vi "ShooterSpeedRegulateV1.vi"(0 "Shooter Speed":T1(ring)) -> (4 "ALL GOOD":bool, 10 "Motor 1 Output":dbl)   [LabVIEW 2012]
uses:
  Robot Global Data.vi
  Max'sToolKit/ConvertVoltageToPercentVbs.vi
  <vilib>/addons/control/pid/pid.llb/PID (DBL).vi
  <vilib>/addons/control/pid/NI_PID_pid.lvlib
panel:
  in  "Reset Shooter PID":bool
  out "Loop Rate (Hz)":dbl
  out "Array Index":dbl
  out "Wheel 1 RPS":dbl
  out "W1 Target RPS":dbl
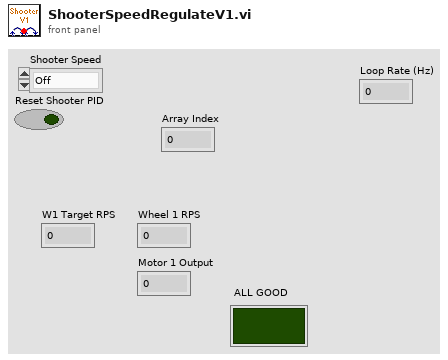
[diagram p1: front panel]
types:
  T1 = enum16{"Off", "2pt Key Shot", "3pt Key Shot", "Back Shot", "Fender Shot", "Key Close", "Key Far"}
  T2 = typedef "WPI_EncoderDevRef.ctl" = cluster{"DevStatus":errorcluster, "EncoderIndex":T3, "CounterIndex":T4, "DistancePerCount":dbl, "Decoding Type":T5}
  T3 = typedef "FPGA_EncoderIdx.ctl" = enum8{"Enc 0", "Enc 1", "Enc 2", "Enc 3", "Invalid"}
  T4 = typedef "FPGA_CounterCtrSystemIndex.ctl" = enum8{"Ctr 0", "Ctr 1", "Ctr 2", "Ctr 3", "Ctr 4", "Ctr 5", "Ctr 6", "Ctr 7", "Invalid"}
  T5 = typedef "WPI_EncoderType.ctl" = enum16{"1x", "2x", "4x"}
  T6 = cluster{"proportional gain (Kc)":dbl, "integral time (Ti, min)":dbl, "derivative time (Td, min)":dbl}
  T7 = typedef "WPI_MotorControlDeviceRef.ctl" = cluster{"DeviceStatus":errorcluster, "Type":enum16{"PWM", "CAN"}, "PWM":cluster{"Digital Module":T8, "PWM Channel":T9, "DeadBand":T10}, "CAN":cluster{"Device Number":u8, "Control Mode":T11, "Semaphore":T12, "Max Vout":dbl}, "Invert":bool, "TransformRef":T13, "InvTransformRef":T13}
  T8 = typedef "FPGA_TypedefDigitalModule.ctl" = enum16{"Digital Module 1", "Digital Module 2"}
  T9 = typedef "FPGA_DIOPWMChannel.ctl" = enum8{"PWM 1", "PWM 2", "PWM 3", "PWM 4", "PWM 5", "PWM 6", "PWM 7", "PWM 8", "PWM 9", "PWM 10", "Invalid"}
  T10 = typedef "WPI_PWMDeadband.ctl" = cluster{"Name":string, "maxPositivePwm":i32, "minPositivePwm":i32, "centerPwm":i32, "maxNegativePwm":i32, "minNegativePwm":i32, "angularRange":u16}
  T11 = typedef "WPI_CANJaguar_ControlMode.ctl" = enum8{"Percent VBus", "Current", "Speed", "Position", "Voltage"}
  T12 = typedef "Semaphore RefNum" = refnum<k1>
  T13 = typedef "WPI_PWMTransform_ConPane.ctl" = refnum<vi>
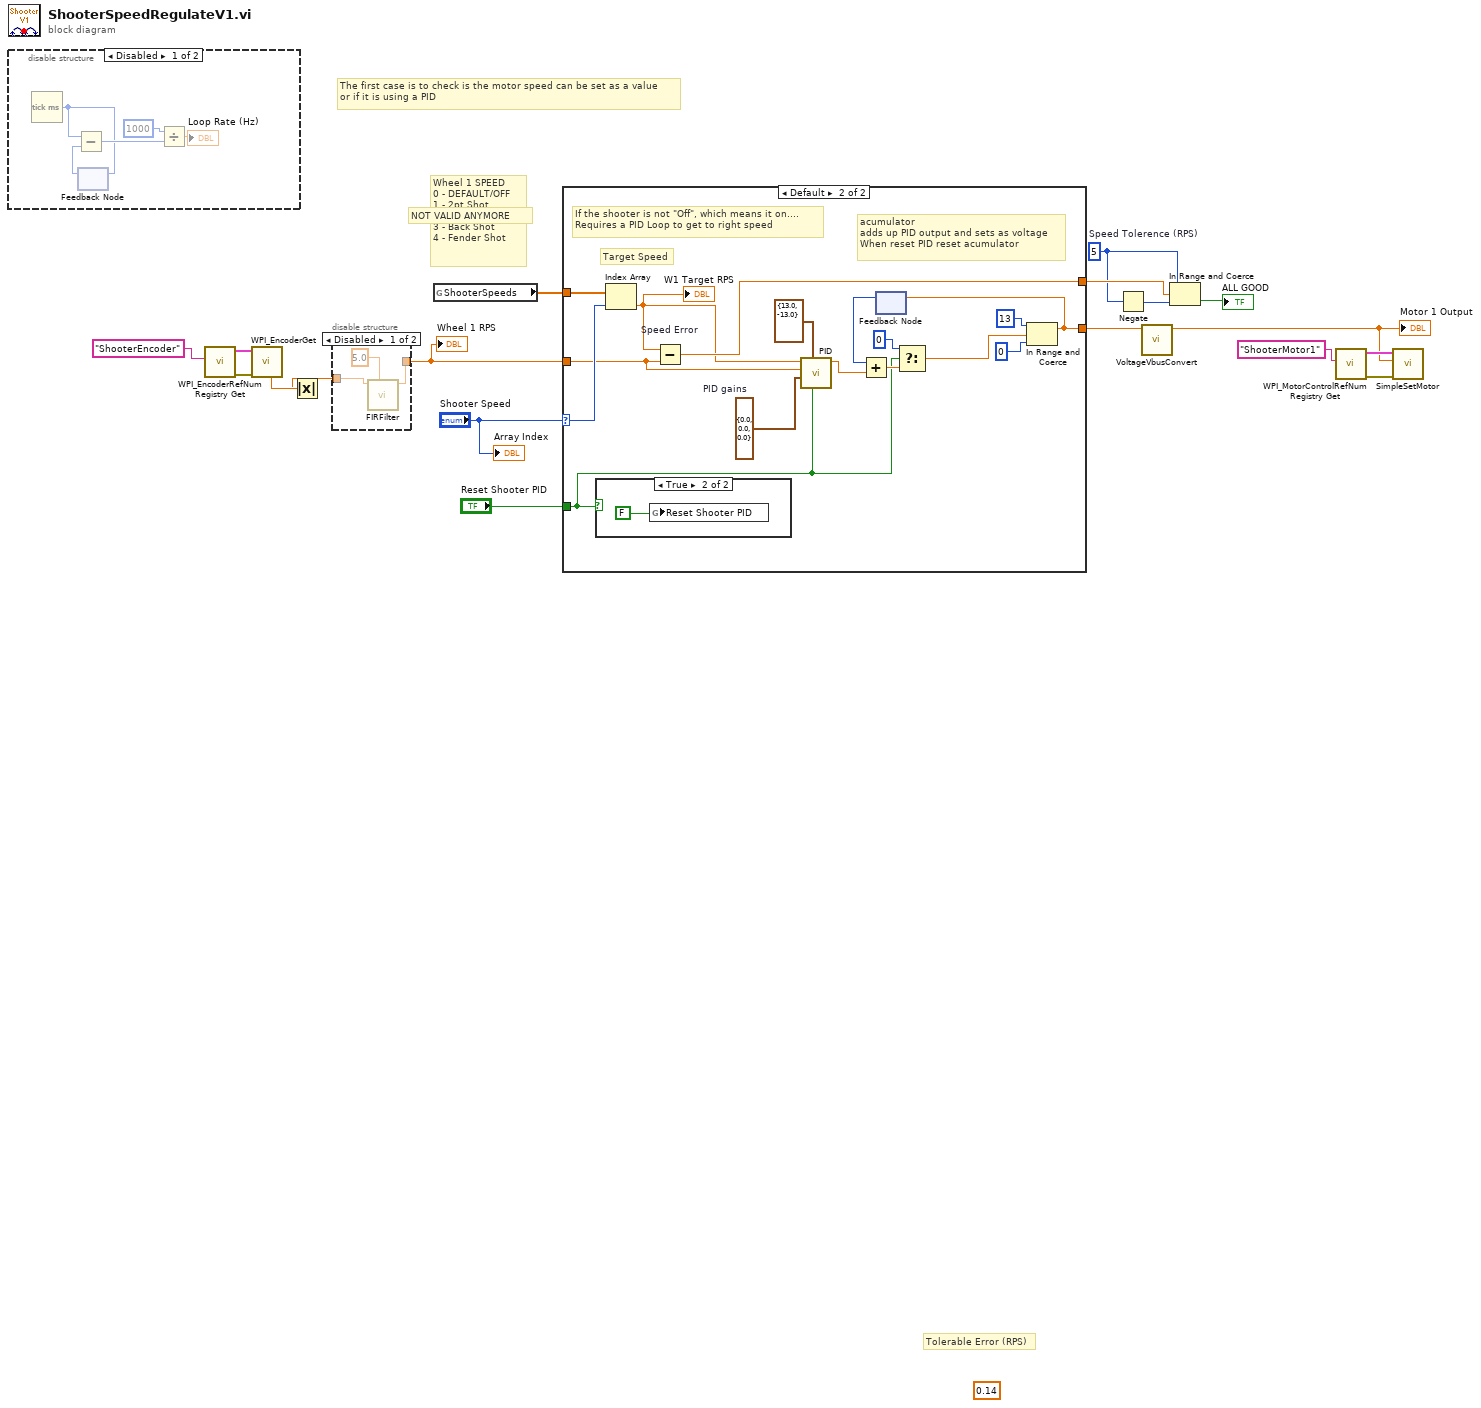
[diagram p0: block diagram]
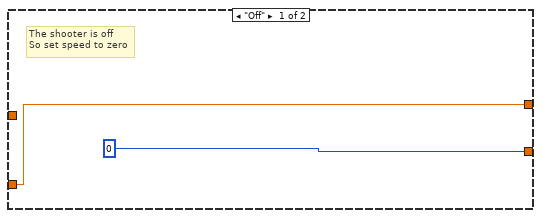
[diagram p4: hidden frame]
diagram:
  w3 = 5  # Speed Tolerence (RPS)
  (unwired) 0.14
  # "NOT VALID ANYMORE"
  # "The first case is to check is the motor speed can be set as a value\nor if it is using a PID"
  # "Tolerable Error (RPS)"
  # "Wheel 1 SPEED\n0 - DEFAULT/OFF\n1 - 2pt Shot\n2 - 3pt Key Shot\n3 - Back Shot\n4 - Fender Shot"
  n1 = disable-structure shown="Disabled" {
    frame Disabled {
      n2 = Tick Count (ms)() -> (millisecond timer value=w19:u32)
      n3 = feedback #1() -> (w20:u32)  [unwired: 1 in]
      n4 = Subtract(x=w19, y=w20) -> (x-y=w22:u32)
      n5 = feedback-in #1(w19) -> ()
      n6 = Divide(x=1000, y=w22) -> (x/y=→"Loop Rate (Hz)":dbl)
    }
    frame Enabled {
    }
  }
  n7 = call <vilib>:"WPI_EncoderRefNum Registry Get.vi"("refnum name"="ShooterEncoder") -> ("error out"=w10:errorcluster, "EncoderDevRef"=w11:T2)  [unwired: 9 in]
  n8 = call <vilib>:"WPI_EncoderGet.vi"("error in (no error)"=w10, "EncoderDevRef"=w11) -> ("Rate"=w7:dbl)  [unwired: 4 in, 5 out]
  n9 = Absolute Value(x=w7) -> (abs(x)=w6:dbl)
  n10 = disable-structure shown="Disabled" {
    disable-tunnel: [w25 w27] -> w9
    disable-tunnel: w6 -> [w24 w27]
    frame Disabled {
      n11 = call "FIRFilter.vi"("Filter Size"=5.0 ("Filter size"), "Input"=w24) -> ("Output"=w25:dbl)  [unwired: 9 in]
    }
    frame Enabled {
    }
  }
  "Wheel 1 RPS" <- w9
  n12 = global read "Robot Global Data.vi" "ShooterSpeeds"() -> (w8:dbl[])
  n13 = case shown="Default" "Shooter Speed" {
    selector: "Shooter Speed" -> [_ w40]
    tunnel: w9 -> [w28 w38]
    tunnel: [0 w42] -> w2
    tunnel: [w28 w39] -> w13
    tunnel: w8 -> [_ w34]
    tunnel: "Reset Shooter PID" -> [_ w31]
    frame "Off" {
      # "The shooter is off\nSo set speed to zero"
    }
    frame Default {
      w41 = T6 {"proportional gain (Kc)"=0.0, "integral time (Ti, min)"=0.0, "derivative time (Td, min)"=0.0}  # PID gains
      # "acumulator\nadds up PID output and sets as voltage\nWhen reset PID reset acumulator"
      # "Target Speed"
      # "If the shooter is not \"Off\", which means it on....\nRequires a PID Loop to get to right speed"
      n14 = case shown="True" w31 {
        frame False {
        }
        frame True {
          n15 = global write "Robot Global Data.vi" "Reset Shooter PID"(FALSE) -> ()
        }
      }
      n16 = Index Array(array=w34, index=w40) -> (element=w32:dbl)
      "W1 Target RPS" <- w32
      n17 = Subtract "Speed Error"(x=w32, y=w38) -> (x-y=w39:dbl)
      n18 = call-poly <vilib>:"PID.vi"("reinitialize? (F)"=w31, "output range"=cluster{"output high":dbl, "output low":dbl} {"output high"=13.0, "output low"=-13.0}, "PID gains"=w41, "process variable"=w38, "setpoint"=w32) -> ("output"=w30:dbl)  [unwired: 5 in, 1 out]
      n19 = feedback #2() -> (w33:i32)  [unwired: 1 in]
      n20 = Add(x=w33, y=w30) -> (x+y=w36:dbl)
      n21 = Select(t=0, s=w31, f=w36) -> (s? t:f=w35:dbl)
      n22 = In Range and Coerce(upper limit=13, x=w35, lower limit=0 ("upper limit")) -> (coerced(x)=w42:dbl)  [unwired: 1 out]
      n23 = feedback-in #2(w42) -> ()
    }
  }
  n24 = Negate(x=w3) -> (-x=w14:i32)
  n25 = call-poly "VoltageVbusConvert.vi"("Voltage"=w2) -> ("Vbus"=w1:dbl)  [unwired: 10 in]
  "Motor 1 Output" <- w1
  n26 = In Range and Coerce(upper limit=w3, x=w13, lower limit=w14) -> (In Range?=→"ALL GOOD":bool)  [unwired: 1 out]
  n27 = call <vilib>:"WPI_MotorControlRefNum Registry Get.vi"("refnum name"="ShooterMotor1") -> ("error out"=w16:errorcluster, "MotorControlDevRef"=w17:T7)  [unwired: 9 in]
  n28 = call "SimpleSetMotor.vi"("error in (no error)"=w16, "Output"=w1, "MotorControlDevRef"=w17) -> ()  [unwired: 7 in, 2 out]
  "Array Index" <- "Shooter Speed"
